vi "Get Int.vi"(8 "error in (no error)":errorcluster, 11 "IIntByRef in":refnum<class "IIntByRef (DVR).lvclass">) -> (0 "error out":errorcluster, 2 "Int":i32, 3 "IIntByRef out":refnum<class "IIntByRef (DVR).lvclass">)   [LabVIEW 2009, in "IIntByRef (DVR).lvclass"]
uses:
  IIntByRef (DVR).lvclass
  Numeric Test Object.lvclass
  Source/IUnknown Class/IUnknown.lvclass
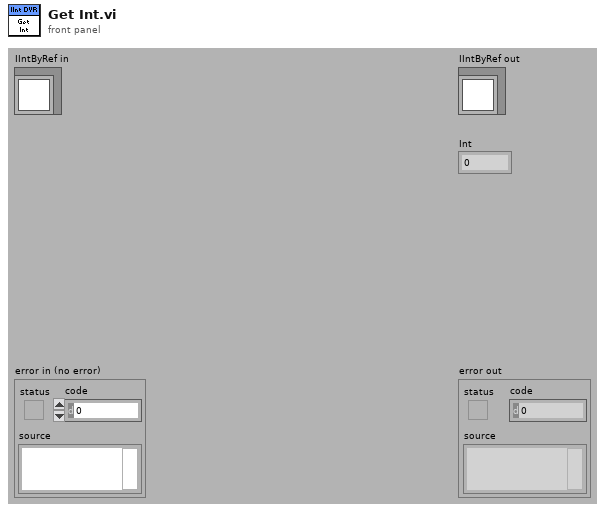
[diagram p1: front panel]
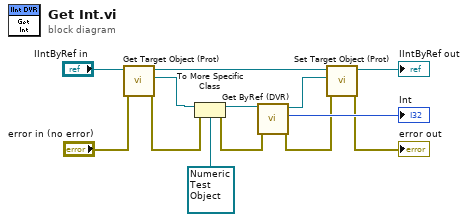
[diagram p0: block diagram]
diagram:
  n1 = call "Get Target Object (Prot).vi"("error in (no error)"="error in (no error)", "IUnknown in"="IIntByRef in") -> ("error out"=w10:errorcluster, "Target Object"=w11:refnum<class "Interfaceable.lvclass">, "IUnknown out"=w4:refnum<class "IIntByRef (DVR).lvclass">)  [unwired: 7 in]
  n2 = To More Specific Class(target class=refnum<class "Numeric Test Object.lvclass"> refnum ("Numeric"), reference=w11, error in=w10) -> (specific class reference=w8:refnum<class "Numeric Test Object.lvclass">, error out=w7:errorcluster)
  n3 = call-dynamic "Get ByRef (DVR).vi"("error in (no error)"=w7, "Numeric in"=w8) -> ("error out"=w2:errorcluster, "Int"=→"Int":i32, "Numeric out"=w5:refnum<class "Numeric Test Object.lvclass">)  [unwired: 7 in]
  n4 = call "Set Target Object (Prot).vi"("error in (no error)"=w2, "Target Object"=w5, "IUnknown in"=w4) -> ("error out"=→"error out":errorcluster, "IUnknown out"=→"IIntByRef out":refnum<class "IIntByRef (DVR).lvclass">)  [unwired: 7 in]
